vi "Wait for Life Cycle State.vi"(8 "error in (no error)":errorcluster, 9 "timeout in ms (-1)":i32=-1, 10 "Lifecycle State":T1, 11 "Process In":refnum<class "Process.lvclass">) -> (0 "error out":errorcluster, 1 "timed out?":bool, 3 "Process Out":refnum<class "Process.lvclass">)   [LabVIEW 2020, in "Process.lvclass"]
doc: "Wait for the process to enter the specified life cycle state."
uses:
  Process.lvclass
  TypeDefs/Lifecycle State.ctl
  Process.lvclass/Process.ctl
  <vilib>/Utility/error.llb/Clear Errors.vi
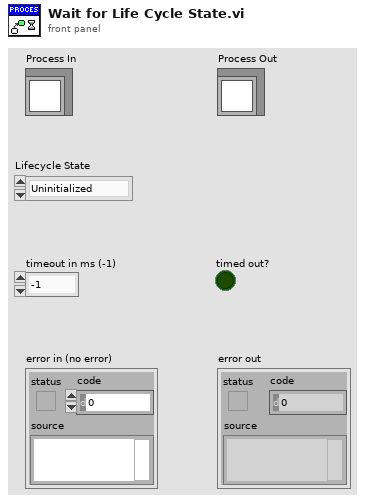
[diagram p1: front panel]
types:
  T1 = typedef "Process.lvclass/Lifecycle State.ctl" = enum16{"Uninitialized", "Initialized", "Started", "Running", "Stopped", "Finished"}
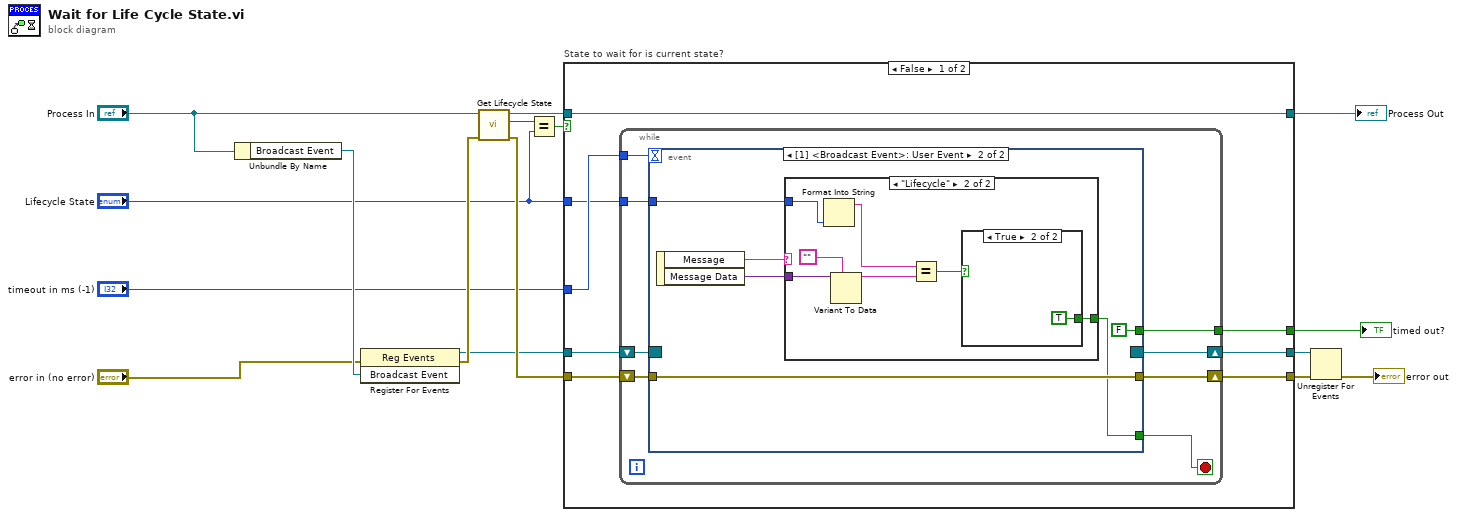
[diagram p0: block diagram]
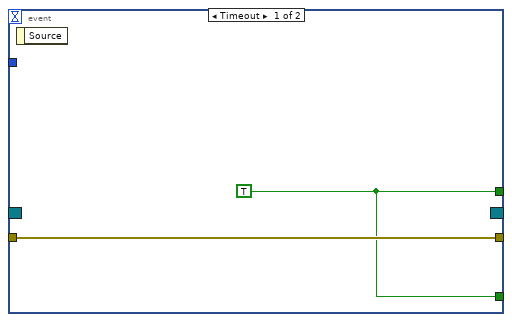
[diagram p2: hidden frame]
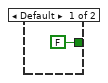
[diagram p3: hidden frame]
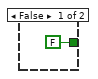
[diagram p4: hidden frame]
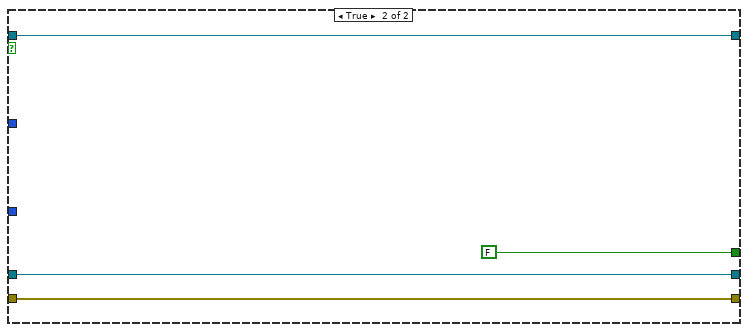
[diagram p5: hidden frame]
diagram:
  n1 = Unbundle By Name("Process In") -> ("Broadcast Event"=w15:refnum<user-event>)
  n2 = register-events(error in="error in (no error)", w15) -> (reference out=w3:refnum<event-registration>, error out=w13:errorcluster)  [unwired: 1 in]
  n3 = call "Get Lifecycle State.vi"("error in (no error)"=w13, "Process In"="Process In") -> ("error out"=w7:errorcluster, "Lifecycle State"=w16:T1, "Process Out"=w9:refnum<class "Process.lvclass">)  [unwired: 6 in, 1 out]
  n4 = Equal?(x=w16, y="Lifecycle State") -> (x = y?=w11:bool)
  n5 = case "State to wait for is current state?" shown="False" w11 {
    tunnel: [w18 w54] -> w10
    tunnel: w9 -> [w18 w54]
    tunnel: [w22 FALSE] -> w8
    tunnel: [w19 w52] -> w6
    tunnel: w7 -> [w20 w52]
    tunnel: [w21 w51] -> w4
    tunnel: w3 -> [w24 w51]
    tunnel: "timeout in ms (-1)" -> [w23 _]
    tunnel: "Lifecycle State" -> [w17 _]
    frame False {
      n6 = while {
        tunnel: w23 -> [w31]
        tunnel: [w30] -> w22
        shift-right: [w29] -> w21
        shift-left: w24 -> [w32]
        shift-right: [w27] -> w19
        shift-left: w20 -> [w28]
        tunnel: w17 -> [w25]
        stop <- w26 stop-if-true
        n7 = event shown="[1] <Broadcast Event>: User Event" {
          selector: w32 -> [_ _]
          dyn-events: [_ _] -> w29
          timeout: w31 -> [_ _]
          tunnel: [w33 FALSE] -> w30
          tunnel: w28 -> [w34 w40]
          tunnel: [w34 w40] -> w27
          tunnel: [w33 w36] -> w26
          tunnel: w25 -> [_ w37]
          event Timeout {
            w33 = TRUE
            n8 = event-data() -> ()  [unwired: 1 in, 1 out]
          }
          event User Event {
            n9 = event-data() -> ("Message"=w39:string, "Message Data"=w38:variant)  [unwired: 1 in]
            n10 = case shown="\"Lifecycle\"" w39 {
              tunnel: w38 -> [_ w48]
              tunnel: w37 -> [_ w46]
              tunnel: [FALSE w42] -> w36
              frame Default {
              }
              frame "Lifecycle" {
                n11 = Format Into String(w46) -> (resulting string=w45:string)  [unwired: 3 in, 1 out]
                n12 = Variant To Data(type="", Variant=w48) -> (data=w44:string)  [unwired: 1 in, 1 out]
                n13 = Equal?(x=w45, y=w44) -> (x = y?=w43:bool)
                n14 = case shown="True" w43 {
                  tunnel: [FALSE TRUE] -> w42
                  frame False {
                  }
                  frame True {
                  }
                }
              }
            }
          }
        }
      }
    }
    frame True {
    }
  }
  "Process Out" <- w10
  "timed out?" <- w8
  n15 = Unregister For Events(event registration refnum=w4, error in=w6) -> (error out=→"error out":errorcluster)
